vi "URI String.vi"(11 "URI in":refnum<class "URI.lvclass">) -> (2 "URI String":string, 3 "URI":refnum<class "URI.lvclass">)   [LabVIEW 2020, in "URI.lvlib" / "URI.lvclass"]
uses:
  URI.lvclass
  URI.lvclass/URI.ctl
  URI.lvlib
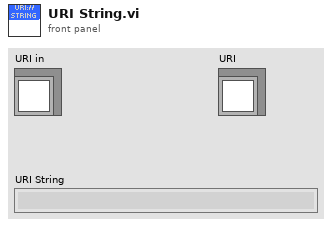
[diagram p1: front panel]
types:
  T1 = typedef "URI.lvlib/URI Components.ctl" = cluster{"Scheme":string, "User Info":string, "Host":string, "Port":string, "Path":string, "Query":string, "Fragment":string}
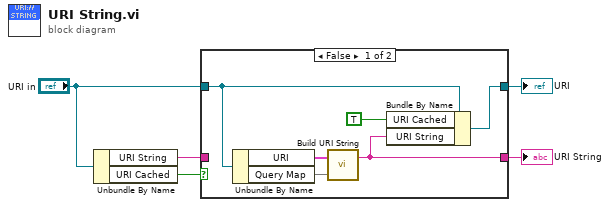
[diagram p0: block diagram]
diagram:
  n1 = Unbundle By Name("URI in") -> ("URI String"=w5:string, "URI Cached"=w3:bool)
  n2 = case shown="False" w3 {
    tunnel: w5 -> [_ w13]
    tunnel: [w8 w13] -> w4
    tunnel: "URI in" -> [w9 w12]
    tunnel: [w6 w12] -> w1
    frame False {
      n3 = Unbundle By Name(w9) -> ("URI"=w11:T1, "Query Map"=w10:map{string, string})
      n4 = call "Build URI String.vi"("URI Components"=w11, "Query Map"=w10) -> ("URI String"=w8:string)  [unwired: 5 in]
      n5 = Bundle By Name(cluster=w9, "URI Cached"=TRUE ("String Cached"), "URI String"=w8) -> (w6:refnum<class "URI.lvclass">)
    }
    frame True {
    }
  }
  "URI String" <- w4
  "URI" <- w1
